vi "setPolarity.vi"(0 "MultiAxisController in":refnum<class "_MultiAxisController.lvclass">, 2 "polarity_items (in)":T2[](array[typedef]), 3 "axis (in)":T1, 5 "error in (no error)":errorcluster) -> (14 "MultiAxisController out":refnum<class "_MultiAxisController.lvclass">, 17 "success?":bool, 18 "response":string, 19 "error out":errorcluster)   [LabVIEW 2013, in "classes.lvlib" / "_MultiAxisController.lvclass"]
doc: "Produced By:\n\n<B>Kod Integrations, LLC</B>\n4835 Marianne Drive\nMount Airy, MD 21771\nhttp://www.kodintegrations.com\nemail: info@kodintegrations.com\nphone: (240) 687-1288"
uses:
  _MultiAxisController.lvclass
  polarity_item.ctl
  polarity.ctl
  axis.ctl
  simple_actions.ctl
  common.lvlib
  _Controller.lvclass
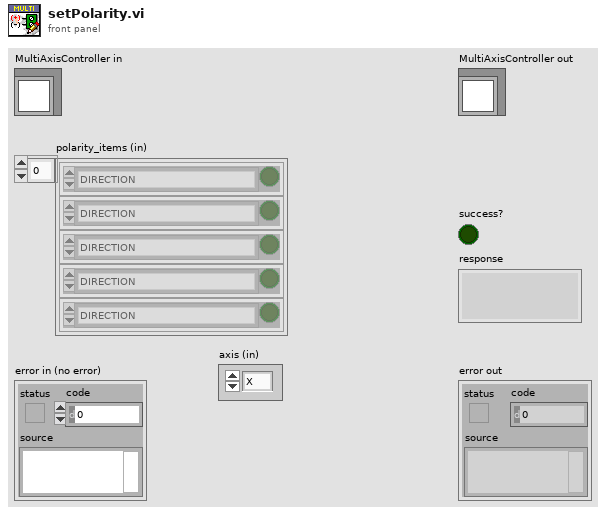
[diagram p1: front panel]
types:
  T1 = typedef "common.lvlib/axis.ctl" = enum16{"X", "Y", "Z", "U"}
  T2 = typedef "common.lvlib/polarity_item.ctl" = cluster{"item":T3, "status":bool}
  T3 = typedef "common.lvlib/polarity.ctl" = enum16{"DIRECTION", "LIMIT", "HOME", "DIG_OUT", "DIG_IN", "ENABLE_OUT", "JUMP_ERR", "LATCH", "Z-CHAN_INDEX", "ENCODER_DECODING:1X", "ENCODER_DECODING:2X", "ENCODER_DECODING:4X", "ALARM", "STANDALONE_ERR", "-", "<reserved/nc>"}
  T4 = typedef "common.lvlib/simple_actions.ctl" = enum16{"from_value", "to_value"}
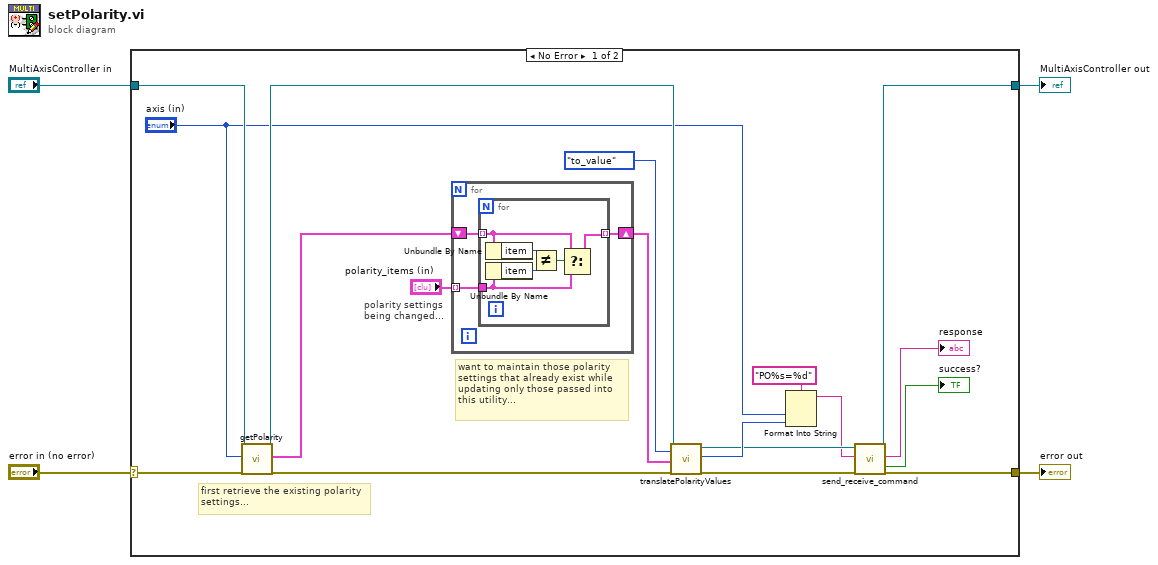
[diagram p0: block diagram]
diagram:
  n1 = case shown="No Error" "error in (no error)" {
    selector: "error in (no error)" -> [w21 w33]
    tunnel: [w13 w33] -> w3
    tunnel: [w8 w32] -> w1
    tunnel: "MultiAxisController in" -> [w22 w32]
    frame No Error {
      # "want to maintain those polarity\nsettings that already exist while\nupdating only those passed into\nthis utility..."
      # "first retrieve the existing polarity\nsettings..."
      # "polarity settings\nbeing changed..."
      n2 = call-dynamic "getPolarity.vi"("MultiAxisController in"=w22, "axis (in)"="axis (in)", "error in (no error)"=w21) -> ("MultiAxisController out"=w16:refnum<class "_MultiAxisController.lvclass">, "polarity_items (out)"=w20:T2[], "error out"=w15:errorcluster)  [unwired: 14 in]
      n3 = for {
        tunnel: "polarity_items (in)" -> [w24] mode=indexing
        shift-right: [w23] -> w18
        shift-left: w20 -> [w25]
        n4 = for {
          tunnel: w25 -> [w28] mode=indexing
          tunnel: w24 -> [w27]
          tunnel: [w26] -> w23 mode=indexing
          n5 = Unbundle By Name(w28) -> ("item"=w31:T3)
          n6 = Unbundle By Name(w27) -> ("item"=w30:T3)
          n7 = Not Equal?(x=w31, y=w30) -> (x != y?=w29:bool)
          n8 = Select(t=w28, s=w29, f=w27) -> (s? t:f=w26:T2)
        }
      }
      n9 = call-dynamic "translatePolarityValues.vi"("Controller in"=w16, "simple_actions"=simple_actions."to_value", "polarity_items (in)"=w18, "error in (no error)"=w15) -> ("Controller out"=w9:refnum<class "_MultiAxisController.lvclass">, "polarity_value (out)"=w10:u32, "error out"=w14:errorcluster)  [unwired: 12 in, 1 out]
      n10 = Format Into String(format string="PO%s=%d", "axis (in)", w10) -> (resulting string=w7:string)  [unwired: 2 in, 1 out]
      n11 = call "send_receive_command.vi"("reference (in)"=w9, "ASCII Command (in)"=w7, "error in (no error)"=w14) -> ("reference (out)"=w8:refnum<class "_MultiAxisController.lvclass">, "response (out)"=→"response":string, "success?"=→"success?":bool, "error out"=w13:errorcluster)  [unwired: 12 in, 1 out]
    }
    frame Error {
    }
  }
  "error out" <- w3
  "MultiAxisController out" <- w1
